vi "Test Load Action.vi"() -> ()   [LabVIEW 2020]
uses:
  neg-pkg/Action/Action.lvclass
panel:
  out "error out":errorcluster
  in  "Args":string[](array[string])
  in  "Action Name":string="install"
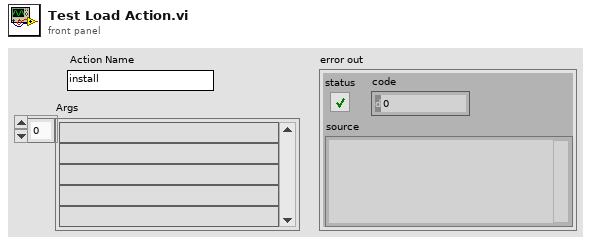
[diagram p1: front panel]
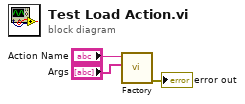
[diagram p0: block diagram]
diagram:
  n1 = call "Factory.vi"("Args"="Args", "Action Name"="Action Name") -> ("error out"=→"error out":errorcluster)  [unwired: 8 in, 1 out]
